vi "Zero_Offset_Channel_Names.vi"() -> (0 "Channel names":string[](array[string]))   [LabVIEW 2017]
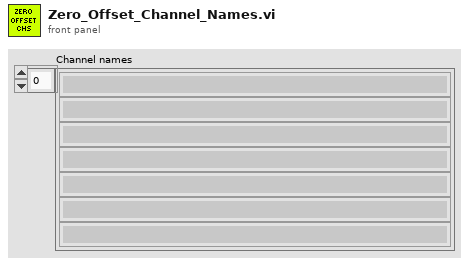
[diagram p1: front panel]
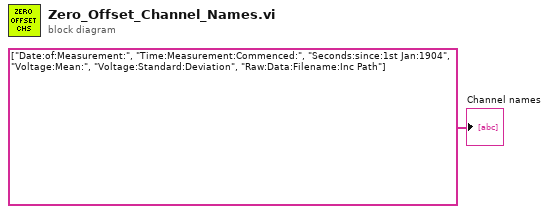
[diagram p0: block diagram]
diagram:
  "Channel names" <- string[] ["Date:of:Measurement:", "Time:Measurement:Commenced:", "Seconds:since:1st Jan:1904", "Voltage:Mean:", "Voltage:Standard:Deviation", "Raw:Data:Filename:Inc Path"] ("Channel names")
